vi "Valid Local File Path Only.vi"(8 "error in":errorcluster, 9 "pattern (*.txt)":string caption="pattern (all files)", 10 "Directory ref":string="Archive Directory", 11 "Path input":path) -> (0 "error out":errorcluster, 3 "Path output":path)   [LabVIEW 2010]
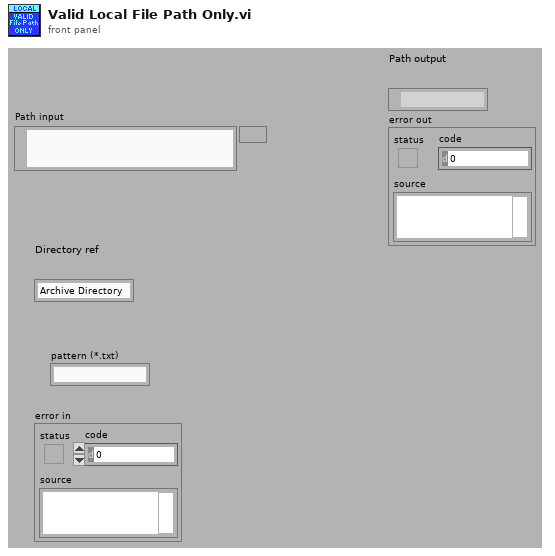
[diagram p1: front panel]
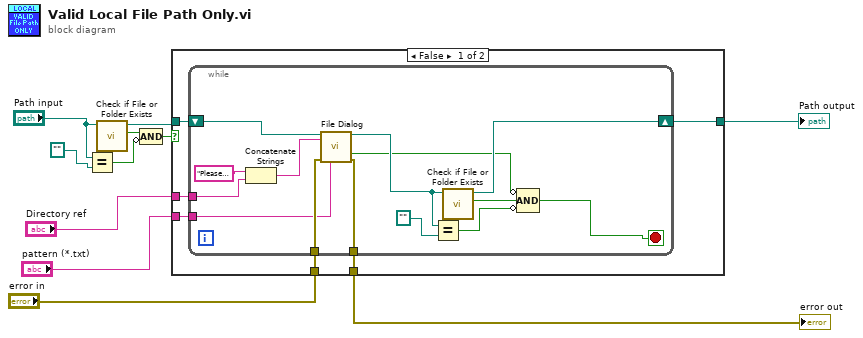
[diagram p0: block diagram]
diagram:
  n1 = Equal?(x="Path input", y=path "") -> (x = y?=w8:bool)
  n2 = call <vilib>:"Check if File or Folder Exists.vi"("path"="Path input") -> ("file or folder exists?"=w7:bool, "dup path"=w10:path)  [unwired: 8 in, 1 out]
  n3 = Compound Arithmetic op=AND(w7, invert w8) -> (w9:bool)
  n4 = case shown="False" w9 {
    tunnel: w10 -> [w17 w33]
    tunnel: [w15 w33] -> w4
    tunnel: "Directory ref" -> [w16 _]
    tunnel: "error in" -> [w14 w32]
    tunnel: [w13 w32] -> w2
    tunnel: "pattern (*.txt)" -> [w12 _]
    frame False {
      n5 = while {
        tunnel: w16 -> [w28]
        shift-right: [w23] -> w15
        shift-left: w17 -> [w31]
        tunnel: w14 -> [w20]
        tunnel: [w19] -> w13
        tunnel: w12 -> [w18]
        stop <- w21 stop-if-true
        n6 = Concatenate Strings("Please specify a Valid File Path for :" ("prompt"), w28) -> (w30:string)
        n7 = call "File Dialog"("start path"=w31, "prompt"=w30, "error in"=w20, "pattern (all files)"=w18) -> ("selected path"=w24:path, "cancelled"=w22:bool, "error out"=w19:errorcluster)  [unwired: 8 in, 1 out]
        n8 = Equal?(x=w24, y=path "") -> (x = y?=w27:bool)
        n9 = call <vilib>:"Check if File or Folder Exists.vi"("path"=w24) -> ("file or folder exists?"=w26:bool, "dup path"=w23:path)  [unwired: 8 in, 1 out]
        n10 = Compound Arithmetic op=AND(invert w22, w26, invert w27) -> (w21:bool)
      }
    }
    frame True {
    }
  }
  "Path output" <- w4
  "error out" <- w2
